vi "AVS_SetSyncMode.vi"(0 "a_hDevice":i32, 7 "a_Enable":u8) -> (4 "Output Value":i32)   [LabVIEW 2009]
uses:
  avaspecx64.dll
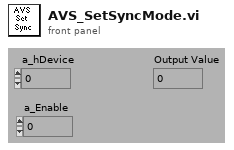
[diagram p1: front panel]
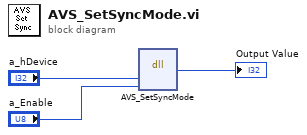
[diagram p0: block diagram]
diagram:
  n1 = dll-call lib="E:/Documents and Settings/mattc/Libraries/Avaspec_Library/trunk/demo_64bit/LabView/LabViewSingleChan/avaspecx64.dll" fn="AVS_SetSyncMode"("a_hDevice"="a_hDevice", "a_Enable"="a_Enable") -> ("return type"=→"Output Value":i32)  [unwired: 5 in, 2 out]
